vi "ChangeUnits00.vi"() -> ()   [LabVIEW 2011]
panel:
  in  "error":errorcluster
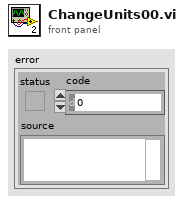
[diagram p1: front panel]
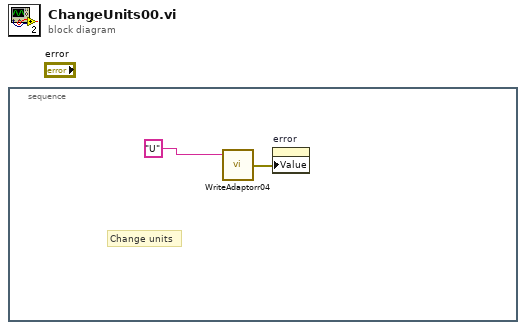
[diagram p0: block diagram]
diagram:
  n1 = stacked-sequence {
    frame #0 {
      # "Change units"
      n2 = call "WriteAdaptorr04.vi"("string to write"="U") -> ("error out"=w1:errorcluster)  [unwired: 2 in]
      n3 = property on="error" class="Clust (strict)"("Value"=w1) -> ()  [unwired: 2 in, 2 out]
    }
  }
